vi "Periodic Tasks.vi"(8 "error in":errorcluster) -> ()   [LabVIEW 2014]
doc: "This VI runs in parallel to other tasks. It can contain as many user-defined periodic loops as you need. These can carry out PID or other sorts of timed response."
uses:
  <vilib>/Rock Robotics/WPI/Solenoid/WPI_SolenoidValue.ctl
  navx-mxp/labview/navX-MXP Library/COMMON/TypeDefs/Data TypeDefs/navX Board Information.ctl
  navx-mxp/labview/navX-MXP Library/COMMON/TypeDefs/Value TypeDefs/navX NAVX_BOARD_CAPABILITY.ctl
  navx-mxp/labview/navX-MXP Library/COMMON/TypeDefs/Value TypeDefs/navX NAVX_BOARD_YAW_AXIS.ctl
  navx-mxp/labview/navX-MXP Library/COMMON/TypeDefs/Data TypeDefs/navX Status Data.ctl
  navx-mxp/labview/navX-MXP Library/COMMON/TypeDefs/Value TypeDefs/navX NAVX_OP_STATUS.ctl
  navx-mxp/labview/navX-MXP Library/COMMON/TypeDefs/Value TypeDefs/navX NAVX_CAL_STATUS.ctl
  navx-mxp/labview/navX-MXP Library/COMMON/TypeDefs/Value TypeDefs/navX NAVX_SENSOR_STATUS.ctl
  navx-mxp/labview/navX-MXP Library/COMMON/TypeDefs/Data TypeDefs/navX Vector Data.ctl
  navx-mxp/labview/navX-MXP Library/COMMON/TypeDefs/Data TypeDefs/navX Quaternion Data.ctl
  navx-mxp/labview/navX-MXP Library/COMMON/TypeDefs/Data TypeDefs/navX YPRH Data.ctl
  <vilib>/Rock Robotics/WPI/CAN/TalonSRX/WPI_CANTalonSRX_GlobalStatus.ctl
  <vilib>/Rock Robotics/WPI/RobotDrive/WPI_RobotDriveGetSetRefNum.vi
  <vilib>/Rock Robotics/WPI/Joystick/WPI_JoystickGetSetRefNum.vi
  <vilib>/Rock Robotics/WPI/Solenoid/WPI_SolenoidSetEnum.vi
  navx-mxp/labview/navX-MXP Library/navX-MXP IMU.lvlib
panel:
  out "element 4":T1
  out "element 3":T1
  out "element 2":T1
  out "element":T1
  out "YPRH":T2
  out "Quaternion":T3
  out "Linear Acceleration":T4
  out "Fused Heading":dbl
  out "Displacement":T4
  in  "Reset Displacement":bool
  out "Altitude":dbl
  out "Status":T5 {"NAVX_OP_STATUS" items=["INITIALIZING", "SELFTEST_IN_PROGRESS", "ERROR", "IMU_AUTOCAL_IN_PROGRESS", "NORMAL"]; "NAVX_CAL_STATUS" items=["IMU_CAL_STATE_MASK"=3, "IMU_CAL_INPROGRESS"=0, "IMU_CAL_ACCUMULATE"=1, "IMU_CAL_COMPLETE"=2, "MAG_CAL_COMPLETE"=4, "BARO_CAL_COMPLETE"=8]}
  out "MPU Temperature (Centigrade)":dbl
  out "Board Information":T9
  out "Set Solenoid State":T12
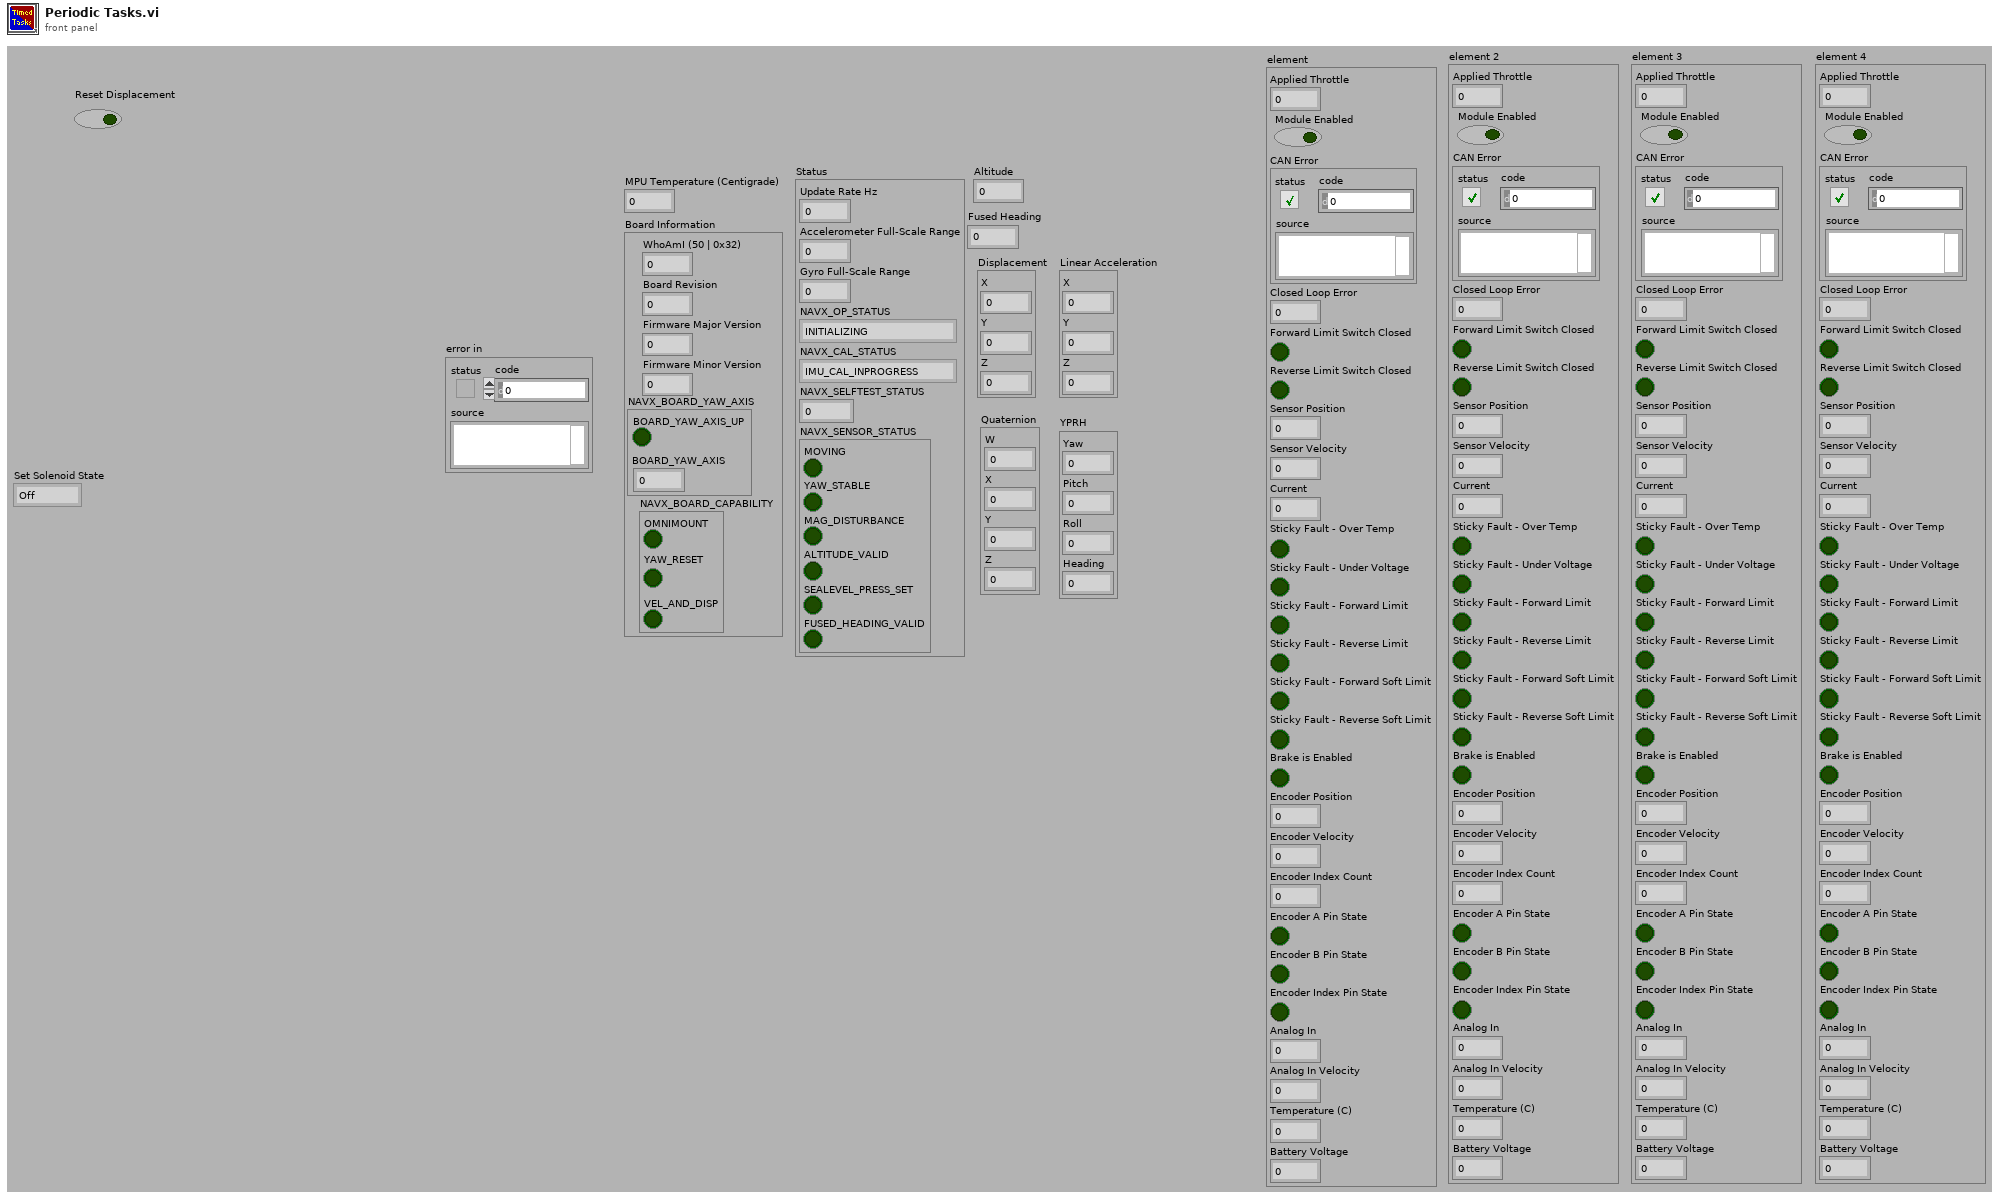
[diagram p1: front panel]
types:
  T1 = typedef "WPI_CANTalonSRX_GlobalStatus.ctl" = cluster{"Applied Throttle":dbl, "Module Enabled":bool, "CAN Error":errorcluster, "Closed Loop Error":dbl, "Forward Limit Switch Closed":bool, "Reverse Limit Switch Closed":bool, "Sensor Position":dbl, "Sensor Velocity":dbl, "Current":dbl, "Sticky Fault - Over Temp":bool, "Sticky Fault - Under Voltage":bool, "Sticky Fault - Forward Limit":bool, "Sticky Fault - Reverse Limit":bool, "Sticky Fault - Forward Soft Limit":bool, "Sticky Fault - Reverse Soft Limit":bool, "Brake is Enabled":bool, "Encoder Position":dbl, "Encoder Velocity":dbl, "Encoder Index Count":dbl, "Encoder A Pin State":bool, "Encoder B Pin State":bool, "Encoder Index Pin State":bool, "Analog In":dbl, "Analog In Velocity":dbl, "Temperature (C)":dbl, "Battery Voltage":dbl}
  T2 = typedef "navX-MXP IMU.lvlib/navX YPRH Data.ctl" = cluster{"Yaw":dbl, "Pitch":dbl, "Roll":dbl, "Heading":dbl}
  T3 = typedef "navX-MXP IMU.lvlib/navX Quaternion Data.ctl" = cluster{"W":dbl, "X":dbl, "Y":dbl, "Z":dbl}
  T4 = typedef "navX-MXP IMU.lvlib/navX Vector Data.ctl" = cluster{"X":dbl, "Y":dbl, "Z":dbl}
  T5 = typedef "navX-MXP IMU.lvlib/navX Status Data.ctl" = cluster{"Update Rate Hz":u8, "Accelerometer Full-Scale Range":u8, "Gyro Full-Scale Range":u16, "NAVX_OP_STATUS":T6, "NAVX_CAL_STATUS":T7, "NAVX_SELFTEST_STATUS":u8, "NAVX_SENSOR_STATUS":T8}
  T6 = typedef "navX-MXP IMU.lvlib/navX NAVX_OP_STATUS.ctl" = u8
  T7 = typedef "navX-MXP IMU.lvlib/navX NAVX_CAL_STATUS.ctl" = u8
  T8 = typedef "navX-MXP IMU.lvlib/navX NAVX_SENSOR_STATUS.ctl" = cluster{"MOVING":bool, "YAW_STABLE":bool, "MAG_DISTURBANCE":bool, "ALTITUDE_VALID":bool, "SEALEVEL_PRESS_SET":bool, "FUSED_HEADING_VALID":bool}
  T9 = typedef "navX-MXP IMU.lvlib/navX Board Information.ctl" = cluster{"WhoAmI (50 | 0x32)":u8, "Board Revision":u8, "Firmware Major Version":u8, "Firmware Minor Version":u8, "NAVX_BOARD_CAPABILITY":T10, "NAVX_BOARD_YAW_AXIS":T11}
  T10 = typedef "navX-MXP IMU.lvlib/navX NAVX_BOARD_CAPABILITY.ctl" = cluster{"OMNIMOUNT":bool, "YAW_RESET":bool, "VEL_AND_DISP":bool}
  T11 = typedef "navX-MXP IMU.lvlib/navX NAVX_BOARD_YAW_AXIS.ctl" = cluster{"BOARD_YAW_AXIS_UP":bool, "BOARD_YAW_AXIS":u8}
  T12 = typedef "WPI_SolenoidValue.ctl" = enum16{"Off", "On", "Forward", "Reverse"}
  T13 = typedef "WPI_RobotDriveDevRef.ctl" = cluster{"DevStatus":errorcluster, "Motors[]":T14[], "Square Inputs":bool, "Max Output":dbl}
  T14 = typedef "WPI_MotorControlDeviceRef.ctl" = cluster{"DeviceStatus":errorcluster, "Type":T15, "PWM":cluster{"Controller":T16, "PWM Channel":T17, "DeadBand":T18}, "CAN":cluster{"Device Number":u8, "Control Mode":T19, "Semaphore":T20, "Max Vout":dbl, "TalonSRX Control Mode":T21}, "Invert":bool, "TransformRef":T22, "InvTransformRef":T22}
  T15 = typedef "WPI_MotorControlType.ctl" = enum16{"PWM", "CAN", "CANTalonSRX"}
  T16 = typedef "FPGA_TypedefDigitalModule.ctl" = enum16{"Controller 1"}
  T17 = typedef "FPGA_DIOPWMChannel.ctl" = enum8{"PWM 0", "PWM 1", "PWM 2", "PWM 3", "PWM 4", "PWM 5", "PWM 6", "PWM 7", "PWM 8", "PWM 9", "PWM MXP 0", "PWM MXP 1", "PWM MXP 2", "PWM MXP 3", "PWM MXP 4", "PWM MXP 5", "PWM MXP 6", "PWM MXP 7", "PWM MXP 8", "PWM MXP 9", "Invalid"}
  T18 = typedef "WPI_PWMDeadband.ctl" = cluster{"Name":string, "maxPositivePwm":i32, "minPositivePwm":i32, "centerPwm":i32, "maxNegativePwm":i32, "minNegativePwm":i32, "angularRange":u16}
  T19 = typedef "WPI_CANJaguar_ControlMode.ctl" = enum8{"Percent VBus", "Current", "Speed", "Position", "Voltage"}
  T20 = typedef "Semaphore RefNum" = refnum<k1>
  T21 = typedef "WPI_CANTalonSRX_APIControlMode.ctl" = enum8{"Percent VBus", "Speed", "Position", "Slave", "Unchanged / Invalid"}
  T22 = typedef "WPI_PWMTransform_ConPane.ctl" = refnum<vi>
  T23 = typedef "WPI_JoystickDevRef.ctl" = cluster{"Device":T24}
  T24 = typedef "WPI_JoystickDeviceEnum.ctl" = enum16{"USB 0", "USB 1", "USB 2", "USB 3", "USB 4", "USB 5"}
  T25 = typedef "WPI_SolenoidDevRef.ctl" = cluster{"DevStatus":errorcluster, "Pneumatics Control Module":u8, "Forward Solenoid Channel":T26, "Reverse Solenoid Channel":T26}
  T26 = typedef "WPI_SolenoidChannel.ctl" = enum8{"Solenoid 0", "Solenoid 1", "Solenoid 2", "Solenoid 3", "Solenoid 4", "Solenoid 5", "Solenoid 6", "Solenoid 7", "Invalid"}
  T27 = typedef "navX-MXP IMU.lvlib/navX Device TypeDef.ctl" = cluster{"navX Interface Protocol":T28, "navX Interface Protocol TypeDefs":cluster{"SPIDevRef":T29, "I2CDevRef":T31}, "navX System Information":cluster{"Board Information":T9, "Status":T5, "Offsets":T33, "LastSampleTimestamp":dbl, "LastSampleValid":bool}, "navX Common Information":cluster{"Update Rate (4Hz-60Hz)":T34, "refnum name":string, "error":errorcluster, "LastSampleFPGATimestamp":dbl}}
  T28 = typedef "navX-MXP IMU.lvlib/navX Interface Protocol.ctl" = enum16{"SPI", "I2C", "SERIAL"}
  T29 = typedef "WPI_SPIDevRef.ctl" = cluster{"DevStatus":errorcluster, "Handle":i32, "Controller":T16, "SPI Bus":T30}
  T30 = typedef "spi_bus.ctl" = enum16{"SPI On-Board, CS0", "SPI On-Board, CS1", "SPI On-Board, CS2", "SPI On-Board, CS3", "SPI MXP", "Invalid"}
  T31 = typedef "WPI_I2CDevRef.ctl" = cluster{"DevStatus":errorcluster, "Controller":T16, "Device Address":u8, "Handle":i32, "I2C Bus":T32}
  T32 = typedef "i2c_bus.ctl" = enum16{"I2C On-Board", "I2C MXP", "Invalid"}
  T33 = typedef "navX-MXP IMU.lvlib/navX Offsets Data.ctl" = cluster{"Yaw":dbl, "Quat W":dbl, "Quat X":dbl, "Quat Y":dbl, "Quat Z":dbl}
  T34 = typedef "navX-MXP IMU.lvlib/navX Update Rate.ctl" = u8
  T35 = cluster{"JoystickDevRef":T23, "RobotDriveDevRef":T13, "SolenoidDevRef":T25, "navX Device TypeDef":T27}
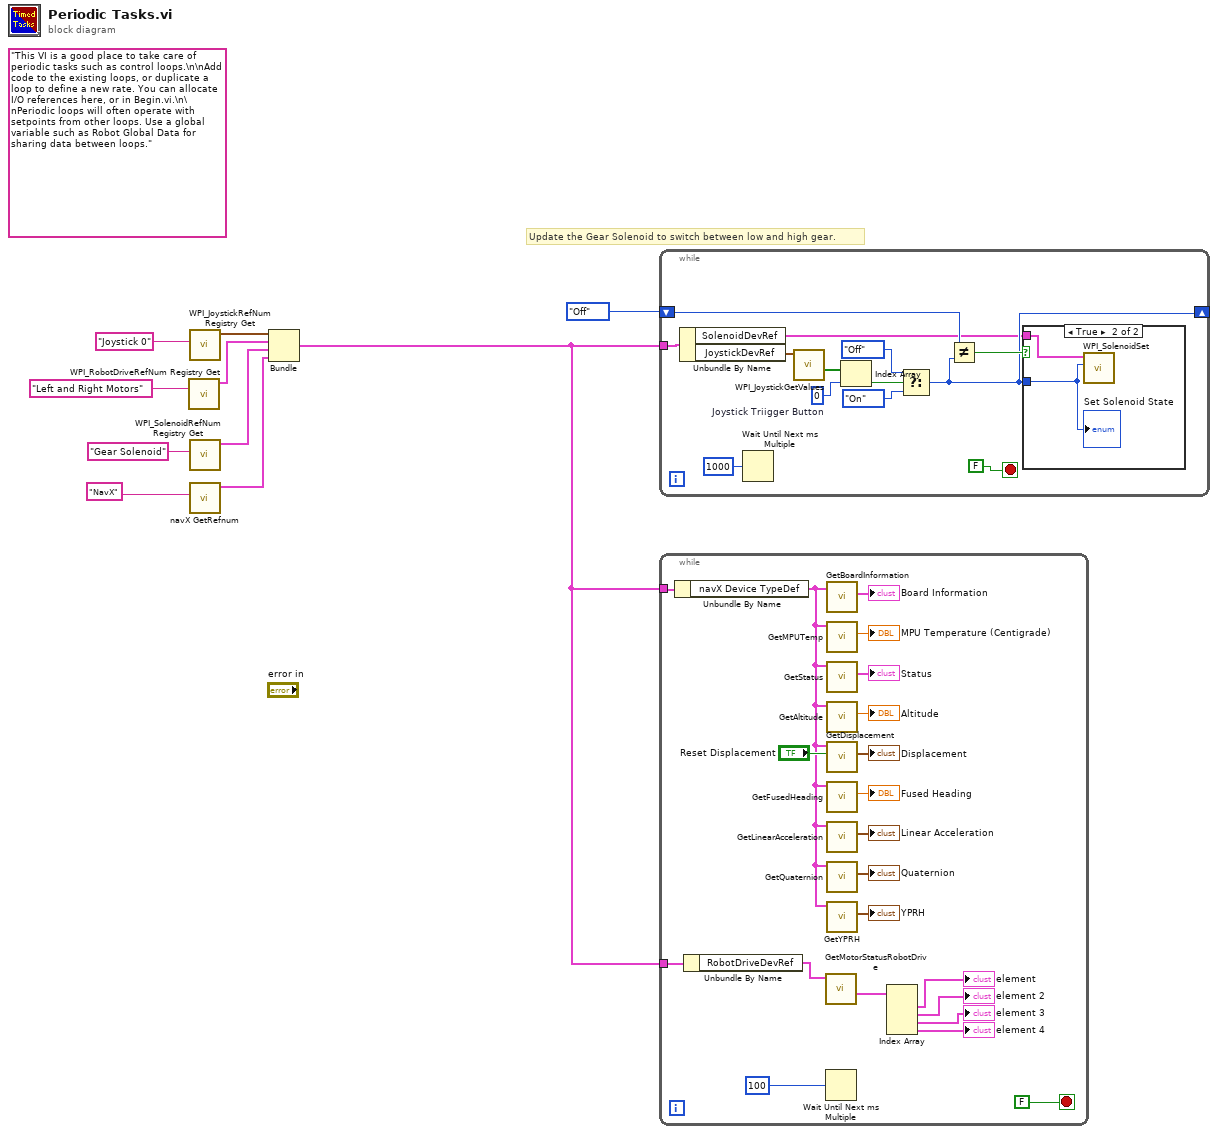
[diagram p0: block diagram]
diagram:
  (unwired) "This VI is a good place to take care of periodic tasks such as control loops.\n\nAdd code to the existing loops, or duplicate a loop to define a new rate. You can allocate I/O references here, or in Begin.vi.\n\nPeriodic loops will often operate with setpoints from other loops. Use a global variable such as Robot Global Data for sharing data between loops."
  # "Update the Gear Solenoid to switch between low and high gear."
  n1 = call <vilib>:"WPI_RobotDriveRefNum Registry Get.vi"("refnum name"="Left and Right Motors") -> ("RobotDriveDevRef"=w8:T13)  [unwired: 1 in, 9 out]
  n2 = call <vilib>:"WPI_JoystickRefNum Registry Get.vi"("refnum name"="Joystick 0") -> ("JoystickDevRef"=w9:T23)  [unwired: 1 in, 9 out]
  n3 = call <vilib>:"WPI_SolenoidRefNum Registry Get.vi"("refnum name"="Gear Solenoid") -> ("SolenoidDevRef"=w5:T25)  [unwired: 9 in, 1 out]
  n4 = call "navX GetRefnum.vi"("refnum name"="NavX") -> ("navX Device TypeDef"=w2:T27)  [unwired: 9 in, 1 out]
  n5 = Bundle("JoystickDevRef"=w9, "RobotDriveDevRef"=w8, "SolenoidDevRef"=w5, "navX Device TypeDef"=w2) -> (w1:T35)  [unwired: 1 out]
  n6 = while {
    tunnel: w1 -> [w19]
    shift-right: [w13] -> _
    shift-left: WPI_SolenoidValue."Off" ("Value") -> [w14]
    stop <- FALSE stop-if-true
    w21 = 0  # Joystick Triigger Button
    n7 = Unbundle By Name(w19) -> ("SolenoidDevRef"=w12:T25, "JoystickDevRef"=w11:T23)
    n8 = Wait Until Next ms Multiple(millisecond multiple=u32 1000) -> ()  [unwired: 1 out]
    n9 = call <vilib>:"WPI_JoystickGetValues.vi"("JoystickDevRef"=w11) -> ("Buttons"=w20:bool[])  [unwired: 6 in, 4 out]
    n10 = Index Array(array=w20, index=w21) -> (element=w18:bool)
    n11 = Select(t=WPI_SolenoidValue."Off" ("Value"), s=w18, f=WPI_SolenoidValue."On" ("Value")) -> (s? t:f=w13:T12)
    n12 = Not Equal?(x=w14, y=w13) -> (x != y?=w15:bool)
    n13 = case shown="True" w15 {
      tunnel: w13 -> [_ w25]
      tunnel: w12 -> [_ w24]
      frame False {
      }
      frame True {
        n14 = call-poly <vilib>:"WPI_SolenoidSet.vi"("Value"=w25, "SolenoidDevRef"=w24) -> ()  [unwired: 8 in, 2 out]
        "Set Solenoid State" <- w25
      }
    }
  }
  n15 = while {
    tunnel: w1 -> [w46]
    tunnel: w1 -> [w32]
    stop <- FALSE stop-if-true
    n16 = Unbundle By Name(w46) -> ("navX Device TypeDef"=w35:T27)
    n17 = Unbundle By Name(w32) -> ("RobotDriveDevRef"=w31:T13)
    n18 = call "GetMotorStatusRobotDrive.vi"("RobotDriveDevRef In"=w31) -> ("Motor Status"=w30:T1[])  [unwired: 9 in, 1 out]
    n19 = Wait Until Next ms Multiple(millisecond multiple=100) -> ()  [unwired: 1 out]
    n20 = call "GetBoardInformation.vi"("navX Device TypeDef"=w35) -> ("Board Information"=→"Board Information":T9)  [unwired: 8 in, 2 out]
    n21 = call "GetMPUTemp.vi"("navX Device TypeDef"=w35) -> ("MPU Temperature (Centigrade)"=→"MPU Temperature (Centigrade)":dbl)  [unwired: 8 in, 2 out]
    n22 = call "GetStatus.vi"("navX Device TypeDef"=w35) -> ("Status"=→"Status":T5)  [unwired: 8 in, 2 out]
    n23 = call "GetAltitude.vi"("navX Device TypeDef"=w35) -> ("Altitude"=→"Altitude":dbl)  [unwired: 8 in, 2 out]
    n24 = call "GetDisplacement.vi"("Reset(F)"="Reset Displacement", "navX Device TypeDef"=w35) -> ("Displacement"=→"Displacement":T4)  [unwired: 6 in, 3 out]
    n25 = call "GetFusedHeading.vi"("navX Device TypeDef"=w35) -> ("Fused Heading"=→"Fused Heading":dbl)  [unwired: 8 in, 2 out]
    n26 = call "GetLinearAcceleration.vi"("navX Device TypeDef"=w35) -> ("Linear Acceleration"=→"Linear Acceleration":T4)  [unwired: 8 in, 2 out]
    n27 = call "GetQuaternion.vi"("navX Device TypeDef"=w35) -> ("Quaternion"=→"Quaternion":T3)  [unwired: 8 in, 2 out]
    n28 = call "GetYPRH.vi"("navX Device TypeDef"=w35) -> ("YPRH"=→"YPRH":T2)  [unwired: 8 in, 2 out]
    n29 = Index Array(array=w30) -> (element #1=→"element":T1, element #2=→"element 2":T1, element #3=→"element 3":T1, element #4=→"element 4":T1)  [unwired: 4 in]
  }
